vi "run-utf.vi"() -> ()   [LabVIEW 2014, in "lv-cli-steps.lvlib"]
uses:
  lv-cli-steps.lvlib
  <vilib>/Utility/error.llb/DialogType.ctl
  <vilib>/NI/UTF Junit Report/utf junit report.lvlib
  <vilib>/Wiresmith Technology/LabVIEW CLI/CLI Class/CLI.lvclass
panel:
  out "error out":errorcluster
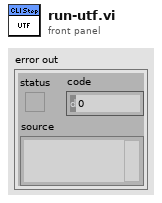
[diagram p1: front panel]
types:
  T1 = typedef "DialogType.ctl" = u16
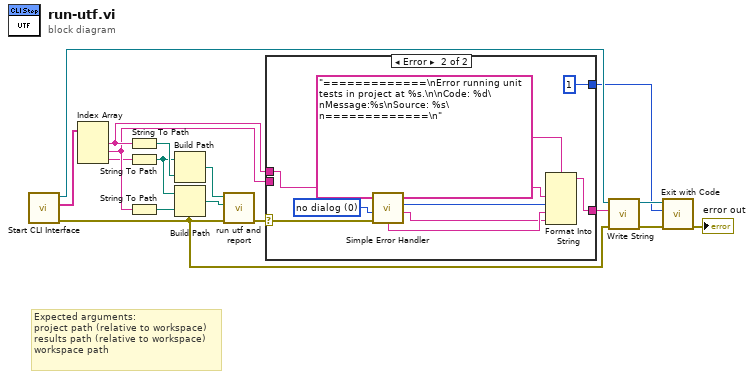
[diagram p0: block diagram]
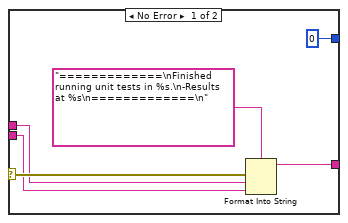
[diagram p2: hidden frame]
diagram:
  # "Expected arguments:\nproject path (relative to workspace)\nresults path (relative to workspace)\nworkspace path"
  n1 = call <vilib>:"Start CLI Interface.vi"() -> ("error out"=w2:errorcluster, "Custom Parameters"=w17:string[], "CLI out"=w13:refnum<class "CLI.lvclass">)  [unwired: 9 in]
  n2 = Index Array(array=w17) -> (element #1=w16:string, element #2=w15:string, element #3=w4:string)  [unwired: 3 in]
  n3 = String To Path(string=w16) -> (path=w9:path)
  n4 = String To Path(string=w4) -> (path=w7:path)
  n5 = String To Path(string=w15) -> (path=w6:path)
  n6 = Build Path(base path=w7, name or relative path=w9) -> (appended path=w8:path)
  n7 = Build Path(base path=w7, name or relative path=w6) -> (appended path=w5:path)
  n8 = call <vilib>:"run utf and report.vi"("error in (no error)"=w2, "junit report file path"=w5, "project file path"=w8) -> ("Error Out"=w1:errorcluster)  [unwired: 8 in]
  n9 = case shown="Error" w1 {
    selector: w1 -> [w22 w31]
    tunnel: w16 -> [w21 w27]
    tunnel: w15 -> [w20 _]
    tunnel: [w19 w32] -> w14
    tunnel: [0 ("Exit Code (0)") 1 ("Exit Code (0)")] -> w10
    frame No Error {
      n10 = Format Into String(format string="=============\nFinished running unit tests in %s.\n-Results at %s\n=============\n", error in=w22, w21, w20) -> (resulting string=w19:string)  [unwired: 1 in, 1 out]
    }
    frame Error {
      w30 = T1 0 items=["no dialog", "OK message", "continue or stop message", "OK message + warnings", "continue/stop + warnings"] ("type of dialog (OK msg:1)")
      n11 = call <vilib>:"Simple Error Handler.vi"("type of dialog (OK msg:1)"=w30, "error in (no error)"=w31) -> ("code out"=w24:i32, "source out"=w25:string, "message"=w26:string)  [unwired: 3 in, 2 out]
      n12 = Format Into String(format string="=============\nError running unit tests in project at %s.\n\nCode: %d\nMessage:%s\nSource: %s\n=============\n", w27, w24, w26, w25) -> (resulting string=w32:string)  [unwired: 2 in, 1 out]
    }
  }
  n13 = call <vilib>:"Write String.vi"("error in (no error)"=w2, "Text to Write"=w14, "CLI in"=w13) -> ("error out"=w12:errorcluster, "CLI out"=w11:refnum<class "CLI.lvclass">)  [unwired: 7 in]
  n14 = call <vilib>:"Exit with Code.vi"("error in (no error)"=w12, "Exit Code (0)"=w10, "CLI in"=w11) -> ("error out"=→"error out":errorcluster)  [unwired: 8 in]
